vi "Test.vi"() -> ()   [LabVIEW 2025]
uses:
  <vilib>/addons/database/NI_Database_API.lvlib
  <vilib>/addons/database/Connection.llb/DB Tools Open Connec (Path).vi
panel:
  out "element":string
  out "index of element":i32
  out "output array":string[](array[string])
  in  "Array":string[][](array[string])
  out "recordset data":variant[][](array[variant])
  in  "Nilai":string
  in  "Combo Box - Dropdown":string(combo)
  out "Hasil Query":string
  out "error out":errorcluster
  in  "Cari":bool
  in  "error in (no error) 2":errorcluster
  out "error in (no error)":errorcluster
  in  "connection information":path
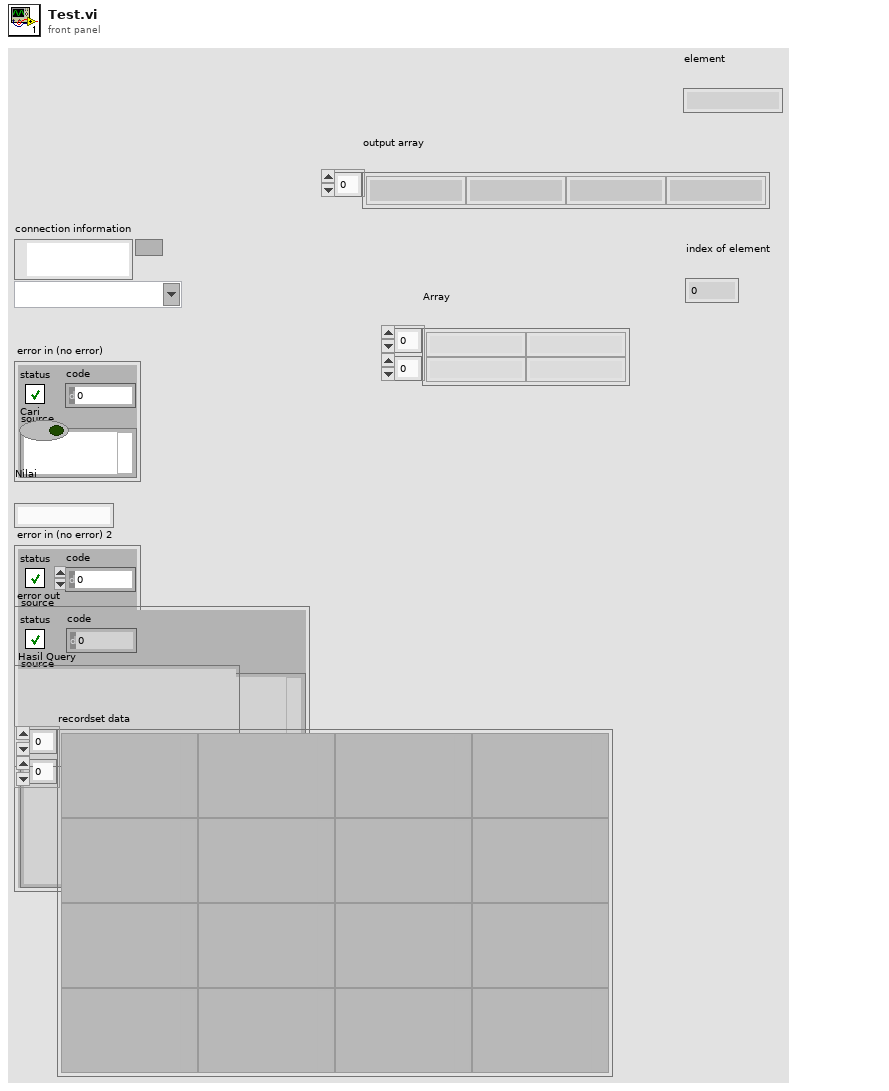
[diagram p1: front panel]
types:
  T1 = typedef "NI_Database_API.lvlib/Conn ObjectReference.ctl" = refnum<k1>
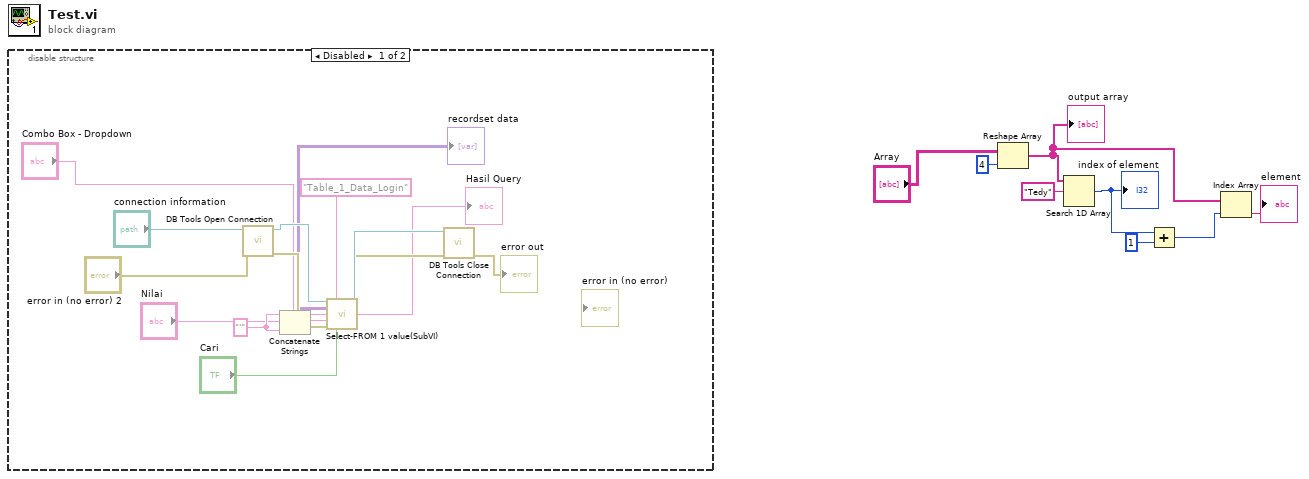
[diagram p0: block diagram]
diagram:
  n1 = disable-structure shown="Disabled" {
    frame Disabled {
      w13 = "'" ("string")
      n2 = call-poly <vilib>:"DB Tools Open Connection.vi"("error in (no error)"="error in (no error) 2", "connection information"="connection information") -> ("error out"=w22:errorcluster, "connection reference"=w23:T1)  [unwired: 6 in]
      n3 = Concatenate Strings(w13, "Nilai", w13) -> (w12:string)
      n4 = call "Select-FROM 1 value(SubVI).vi"("connection reference"=w23, "TABLE"="Table_1_Data_Login", "COLOUM Data"="Combo Box - Dropdown", "Nilainya"=w12, "error in (no error)"=w22, "Cari"="Cari") -> ("connection reference 2"=w18:T1, "recordset data"=→"recordset data":variant[][], "Hasil Query"=→"Hasil Query":string, "error out"=w17:errorcluster)  [unwired: 5 in, 1 out]
      n5 = call <vilib>:"DB Tools Close Connection.vi"("error in (no error)"=w17, "connection reference"=w18) -> ("error out"=→"error out":errorcluster)  [unwired: 5 in]
    }
    frame Enabled {
    }
  }
  n6 = Reshape Array("Array", 4 ("dimension size")) -> (w5:string[])
  "output array" <- w5
  n7 = Search 1D Array(1D array=w5, element="Tedy") -> (index of element=w4:i32)  [unwired: 1 in]
  "index of element" <- w4
  n8 = Add(x=w4, y=1) -> (x+y=w2:i32)
  n9 = Index Array(array=w5, index=w2) -> (element=→"element":string)
